vi "get cluster names.vi"(11 "Variant":variant) -> (3 "Data Labels Array":string[](array[string])=["data a", "data a 2", "data a 3", "data a 4", "data b", "data b 2", "data b 3", "data b 4", "data c", "data d"])   [LabVIEW 2013]
uses:
  <vilib>/Utility/VariantDataType/VariantType.lvlib
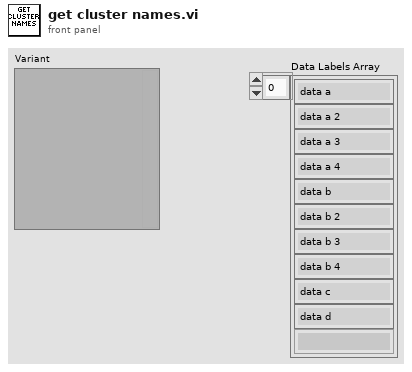
[diagram p1: front panel]
types:
  T1 = typedef "VariantType.lvlib/Type.ctl" = enum8{"Invalid Type", "Void", "I8", "I16", "I32", "I64", "U8", "U16", "U32", "U64", "Single Float", "Double Float", "Extended Float", "Single Complex", "Double Complex", "Extended Complex", "Enum U8", "Enum U16", "Enum U32", "Enum U64", "Single Float With Unit", "Double Float With Unit", "Extended Float With Unit", "Single Complex with Unit", "Double Complex with Unit", "Extended Complex with Unit", "Boolean", "String", "Path", "Picture", "Tag", "Array", "Cluster", "Variant", "LV Variant", "Waveform", "Timestamp", "Digital Waveform", "Digital Data", "ExpressData", "Refnum", "External Data", "VI", "Poly VI", "LabVIEW Class Instance", "Fixed Point"}
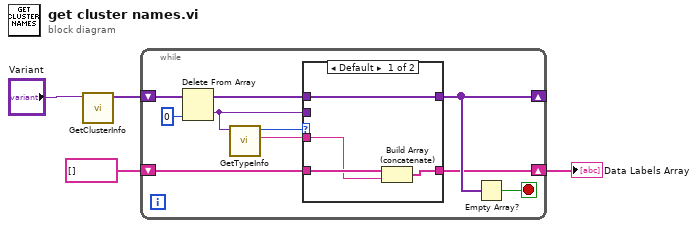
[diagram p0: block diagram]
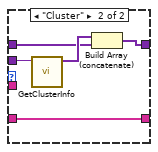
[diagram p2: hidden frame]
diagram:
  n1 = call <vilib>:"GetClusterInfo.vi"("Variant"="Variant") -> ("Cluster Elements"=w4:variant[])  [unwired: 9 in, 1 out]
  n2 = while {
    shift-right: [w8] -> _
    shift-left: w4 -> [w14]
    shift-right: [w6] -> w2
    shift-left: string[] [] -> [w7]
    stop <- w12 stop-if-true
    n3 = Delete From Array(array=w14, index=0) -> (deleted portion=w9:variant, array with subset deleted=w10:variant[])  [unwired: 1 in]
    n4 = call <vilib>:"GetTypeInfo.vi"("Variant"=w9) -> ("Name"=w5:string, "Type Enum"=w11:T1)  [unwired: 6 in, 3 out]
    n5 = case shown="Default" w11 {
      tunnel: w10 -> [w18 w21]
      tunnel: w9 -> [_ w23]
      tunnel: [w18 w20] -> w8
      tunnel: w7 -> [w17 w19]
      tunnel: [w15 w19] -> w6
      tunnel: w5 -> [w16 _]
      frame Default {
        n6 = Build Array (concatenate)(w17, w16) -> (w15:string[])
      }
      frame "Cluster" {
        n7 = call <vilib>:"GetClusterInfo.vi"("Variant"=w23) -> ("Cluster Elements"=w22:variant[])  [unwired: 9 in, 1 out]
        n8 = Build Array (concatenate)(w22, w21) -> (w20:variant[])
      }
    }
    n9 = Empty Array?(array=w8) -> (empty?=w12:bool)
  }
  "Data Labels Array" <- w2
